vi "Copy Set Default Value VI.vi"(11 "error in (no error)":errorcluster) -> (15 "error out":errorcluster)   [LabVIEW 2021, in "Converter.lvlib"]
uses:
  Converter.lvlib
  Path Functions/Path Functions.lvlib
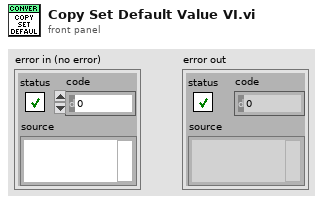
[diagram p1: front panel]
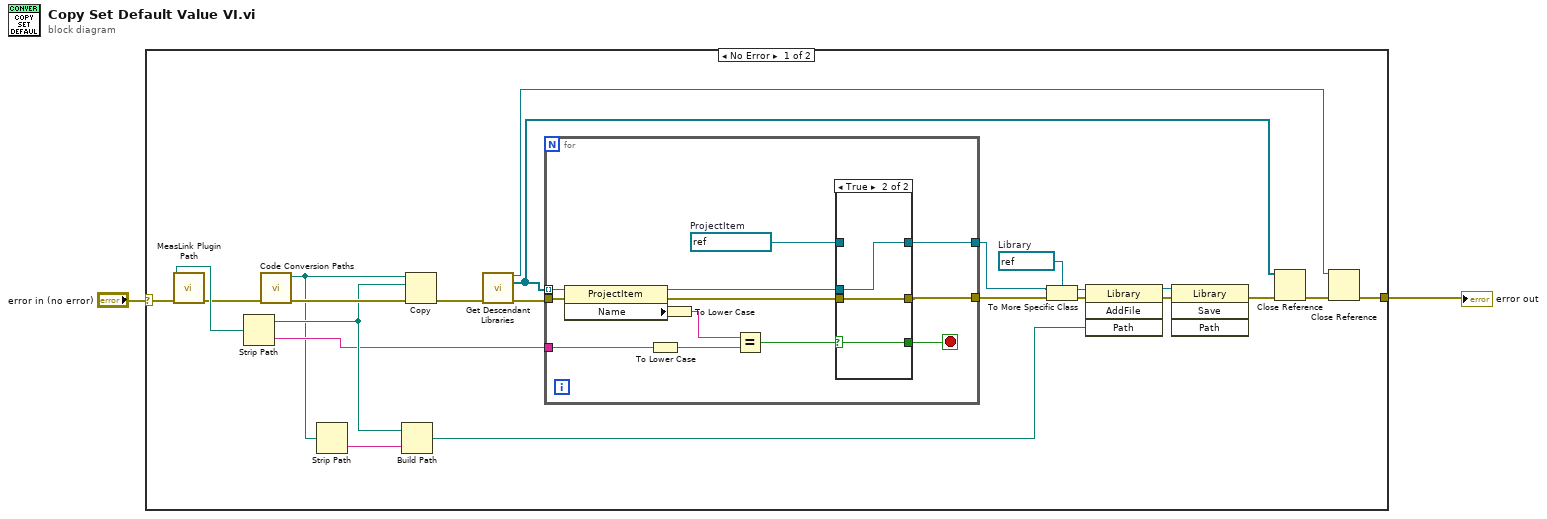
[diagram p0: block diagram]
diagram:
  n1 = case shown="No Error" "error in (no error)" {
    selector: "error in (no error)" -> [w23 w45]
    tunnel: [w5 w45] -> w2
    frame No Error {
      w11 = refnum<vi> refnum  # Library
      n2 = call "MeasLink Plugin Path.vi"("error in (no error)"=w23) -> ("Measurement UI Lib"=w24:path, "error out"=w22:errorcluster)  [unwired: 2 in, 11 out]
      n3 = Strip Path(path=w24) -> (stripped path=w18:path, name=w17:string)
      n4 = call "Code Conversion Paths.vi"("error in (no error)"=w22) -> ("Deafult value setter VI"=w4:path, "error out"=w25:errorcluster)  [unwired: 6 in, 7 out]
      n5 = Strip Path(path=w4) -> (name=w3:string)  [unwired: 1 out]
      n6 = Build Path(base path=w18, name or relative path=w3) -> (appended path=w16:path)
      n7 = Copy(8:w25, 10:w18, 11:w4) -> (0:w21:errorcluster)  [unwired: 2 in, 2 out]
      n8 = call "Get Descendant Libraries.vi"("error in (no error)"=w21) -> ("Project out"=w6:refnum<vi>, "All Descendents"=w15:refnum<vi>[], "error out"=w20:errorcluster)  [unwired: 12 in]
      n9 = for {
        tunnel: w15 -> [w38] mode=indexing
        tunnel: [w31] -> w10
        tunnel: [w30] -> w19
        tunnel: w17 -> [w29]
        tunnel: w20 -> [w28]
        stop <- w32 stop-if-true
        w35 = refnum<vi> refnum  # ProjectItem
        n10 = property class="ProjectItem"(reference=w38, error in=w28) -> (reference out=w34:refnum<vi>, error out=w33:errorcluster, "Name"=w37:string)
        n11 = To Lower Case(string=w29) -> (all lower case string=w26:string)
        n12 = To Lower Case(string=w37) -> (all lower case string=w27:string)
        n13 = Equal?(x=w27, y=w26) -> (x = y?=w36:bool)
        n14 = case shown="True" w36 {
          selector: w36 -> [w40 w43]
          tunnel: w34 -> [_ w44]
          tunnel: [w39 w42] -> w30
          tunnel: [w41 w44] -> w31
          tunnel: w35 -> [w41 _]
          tunnel: [w40 w43] -> w32
          tunnel: w33 -> [w39 w42]
          frame False {
          }
          frame True {
          }
        }
      }
      n15 = To More Specific Class(target class=w11, reference=w10, error in=w19) -> (specific class reference=w9:refnum<vi>, error out=w12:errorcluster)
      n16 = invoke class="Library" method="AddFile"(reference=w9, error in=w12, "Path"=w16) -> (reference out=w13:refnum<vi>, error out=w8:errorcluster)  [unwired: 1 in, 2 out]
      n17 = invoke class="Library" method="Save"(reference=w13, error in=w8) -> (error out=w7:errorcluster)  [unwired: 2 in, 3 out]
      n18 = Close Reference(reference=w15, error in (no error)=w7) -> (error out=w14:errorcluster)
      n19 = Close Reference(reference=w6, error in (no error)=w14) -> (error out=w5:errorcluster)
    }
    frame Error {
    }
  }
  "error out" <- w2
